vi "Find contact statistic.vi"(0 "reference in":refnum<class "Force Curve_tdms.lvclass">, 5 "error in (no error)":errorcluster) -> (14 "reference out":refnum<class "Force Curve_tdms.lvclass">, 16 "contact point index out":i32, 19 "error out":errorcluster)   [LabVIEW 2019, in "Force Curve_tdms.lvclass"]
doc: "Calculates the index of the contact point by getting the mean and median of the approach portion of the Fcurve, based on std.dev*K (constant)"
uses:
  Force Curve_tdms.lvclass
  Signal In.ctl
  <vilib>/Analysis/2dsp.llb/Decimate (single shot, DBL).vi
  <vilib>/Analysis/NI_AALBase.lvlib
  <vilib>/Analysis/NI_AALPro.lvlib
panel:
  out "x+y":dbl
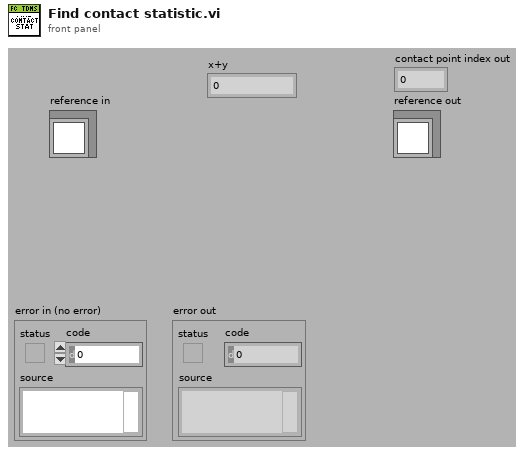
[diagram p1: front panel]
types:
  T1 = typedef "Force Curve_tdms.lvclass/Signal In.ctl" = enum16{"Deflection", "SensorIn", "MockOut", "ZstageOut"}
  T2 = typedef "Force Curve_tdms.lvclass/ObjectAttributes.ctl" = cluster{"MyAttribute":dbl, "Processed data":waveform(dbl)[], "Fcurve Raw Metadata":T3, "Fcurve Metadata":T4, "Fcurve index":T5, "Tau Delay (ms)":dbl, "Contact Spread of dev":dbl, "Fcurve":T6}
  T3 = typedef "TDMS_DataHandler.lvclass/Fcurve Meta data.ctl" = cluster{"property names":string[], "property values":variant[]}
  T4 = typedef "Force Curve_tdms.lvclass/Fcurve Meta data analysis.ctl" = cluster{"dt (us)":dbl, "Dec Factor":dbl, "Z piezo Sensitivity (nm/V)":dbl, "K (N/m)":dbl, "Sp (V)":dbl, "Contact (ms)":dbl, "Zpos contact":dbl, "Vel_app (nm/s)":dbl, "Vel_ret (nm/s)":dbl, "deltaV (nm)":dbl, "Def_V0 (v)":dbl, "Decimating Factor":dbl}
  T5 = typedef "Force Curve_tdms.lvclass/Fcurve Index .ctl" = cluster{"Setpoint index":i32, "Max force index":i32, "Contact point index":i32, "Appoach indices":cluster{"Start":i32, "End":i32}, "Contact indices":cluster{"Start":i32, "End":i32}, "Retract indices":cluster{"Start":i32, "End":i32}}
  T6 = typedef "Force Curve_tdms.lvclass/Force Curve data.ctl" = cluster{"Approach":cluster{"X":dbl[], "Y":dbl[]}, "Contact":cluster{"X":dbl[], "Y":dbl[]}, "Retract":cluster{"X":dbl[], "Y":dbl[]}}
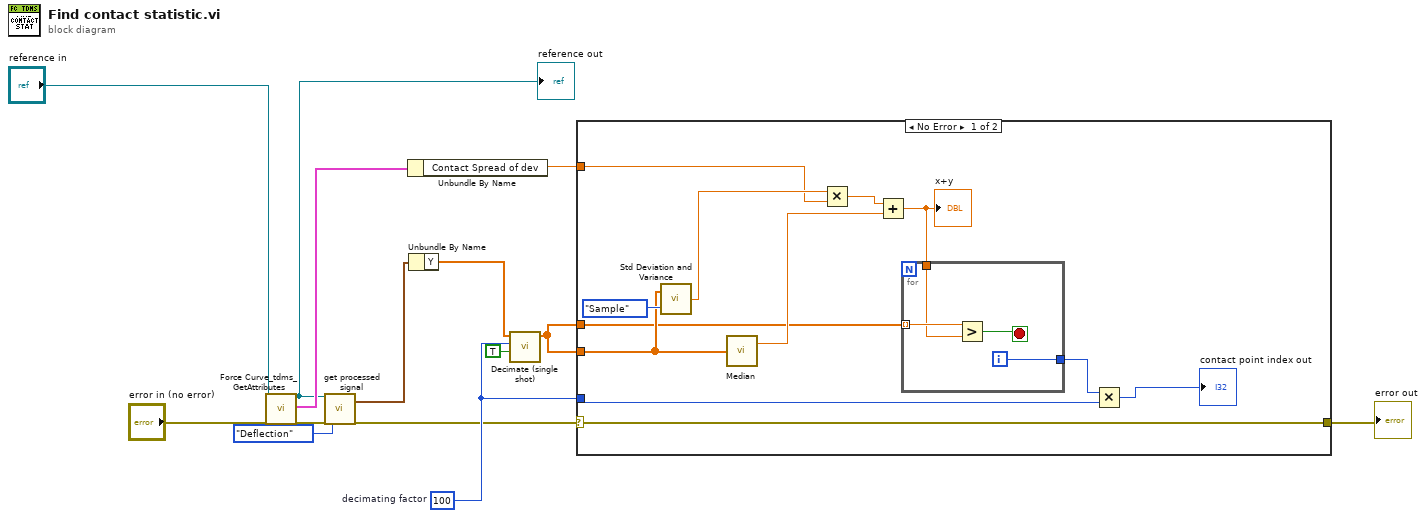
[diagram p0: block diagram]
diagram:
  w13 = 100  # decimating factor
  n1 = call "Force Curve_tdms_GetAttributes.vi"("reference in"="reference in", "error in (no error)"="error in (no error)") -> ("reference out"=w3:refnum<class "Force Curve_tdms.lvclass">, "attributes"=w8:T2, "error out"=w6:errorcluster)  [unwired: 14 in, 1 out]
  "reference out" <- w3
  n2 = call "get processed signal.vi"("reference in"=w3, "error in (no error)"=w6, "Signal in"=Signal_In."Deflection") -> ("Wfm out"=w2:waveform(dbl), "error out"=w5:errorcluster)  [unwired: 14 in, 1 out]
  n3 = Unbundle By Name(w8) -> ("Contact Spread of dev"=w7:dbl)
  n4 = Unbundle By Name(w2) -> ("Y"=w12:dbl[])
  n5 = call-poly <vilib>:"Decimate (single shot).vi"("averaging"=TRUE, "decimating factor"=w13, "X"=w12) -> ("Decimated Array"=w11:dbl[])  [unwired: 7 in, 1 out]
  n6 = case shown="No Error" w5 {
    selector: w5 -> [w26 w31]
    tunnel: [w26 w31] -> w14
    tunnel: w11 -> [w21 _]
    tunnel: w13 -> [w18 _]
    tunnel: w11 -> [w17 _]
    tunnel: w7 -> [w15 _]
    frame No Error {
      n7 = call <vilib>:"Std Deviation and Variance.vi"("X"=w21, "Weighting (Sample)"=enum16{"Sample", "Population"}."Sample") -> ("standard deviation"=w22:dbl)  [unwired: 2 out]
      n8 = call <vilib>:"Median.vi"("X"=w21) -> ("median"=w24:dbl)  [unwired: 1 out]
      n9 = Multiply(x=w22, y=w15) -> (x*y=w23:dbl)
      n10 = Add(x=w23, y=w24) -> (x+y=w20:dbl)
      "x+y" <- w20
      n11 = for {
        tunnel: w17 -> [w30] mode=indexing
        tunnel: w20 -> [w29]
        tunnel: [w27] -> w19
        i -> [w27]
        stop <- w28 stop-if-true
        n12 = Greater?(x=w30, y=w29) -> (0:w28:bool)
      }
      n13 = Multiply(x=w19, y=w18) -> (x*y=→"contact point index out":i32)
    }
    frame Error {
    }
  }
  "error out" <- w14
